vi "Cargo Low Shoot (SubVI).vi"(6 "lowShoot":bool, 9 "desiredIntakePosition":dbl, 10 "desiredIndexerOutput":dbl, 11 "desiredIntakeOutput":dbl) -> (1 "desiredIntakePosition":dbl, 2 "desiredIndexerOutput":dbl, 3 "desiredIntakeOutput":dbl)   [LabVIEW 2020]
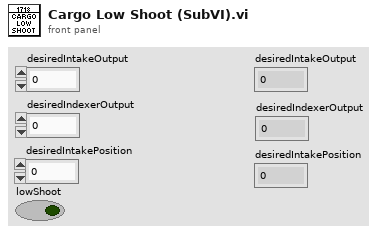
[diagram p1: front panel]
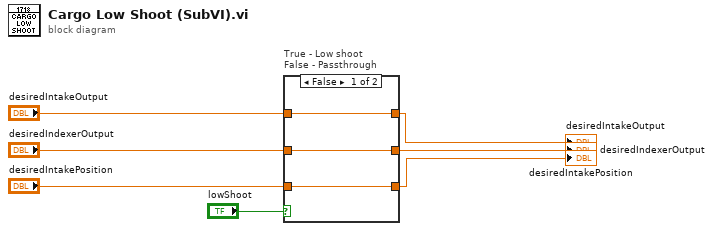
[diagram p0: block diagram]
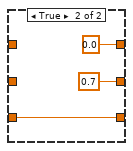
[diagram p2: hidden frame]
diagram:
  n1 = case "True - Low shoot\nFalse - Passthrough" shown="False" "lowShoot" {
    tunnel: "desiredIntakePosition" -> [w8 w11]
    tunnel: "desiredIndexerOutput" -> [w9 _]
    tunnel: "desiredIntakeOutput" -> [w10 _]
    tunnel: [w10 0.0 ("Intake")] -> w5
    tunnel: [w9 0.7 ("Intake")] -> w6
    tunnel: [w8 w11] -> w7
    frame False {
    }
    frame True {
    }
  }
  "desiredIntakePosition" <- w7
  "desiredIndexerOutput" <- w6
  "desiredIntakeOutput" <- w5
